vi "Config Directory.vi"() -> (2 "Config Directory":path)   [LabVIEW 2020, in "File IO.lvlib" / "Project Locations.lvlib"]
doc: "Returns the Config directory for the application, independent of whether it is run with the LabVIEW runtime, as a standalone EXE, using an installer, or during development in LabVIEW."
uses:
  Project Locations.lvlib
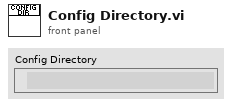
[diagram p1: front panel]
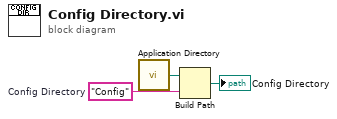
[diagram p0: block diagram]
diagram:
  w2 = "Config"  # Config Directory
  n1 = call <vilib>:"Application Directory.vi"() -> ("Application Directory"=w3:path)
  n2 = Build Path(base path=w3, name or relative path=w2) -> (appended path=→"Config Directory":path)
